vi "AlliGator Update Phasor Ratio Reference.vi"(7 "State Indicators Refnum":refnum<vi>, 8 "error in (no error)":errorcluster, 9 "Lifetime":dbl[unit], 10 "Reference Idx (0 or 1)":i32, 11 "Phasor":cluster{"X":dbl, "Y":dbl}) -> (0 "error out":errorcluster)   [LabVIEW 2021, in "AlliGator Phasor Graph.lvlib"]
doc: "Sets Phasor References status LEDs."
uses:
  AlliGator Phasor Graph.lvlib
  Globals, Variables, Constants/AlliGator Variables List.ctl
  Action Engine/AlliGator State Indicators List.ctl
  Globals, Variables, Constants/AlliGator Globals, Variables & Constants.lvlib
  Action Engine/AlliGator Action Engine.lvlib
  GUI/AlliGator GUI.lvlib
  Settings/AlliGator Settings.lvlib
  Error/Error.lvlib
panel:
  # "see the AlliGator License on the block diagram (Ctrl+E or Window:Show Block Diagram)"
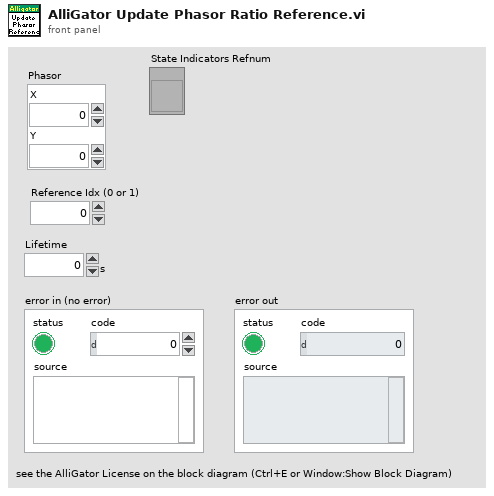
[diagram p1: front panel]
types:
  T1 = typedef "AlliGator Globals, Variables & Constants.lvlib/AlliGator Variables List.ctl" = enum16{"---- GUI ----", "GUI:Initialization Status", "GUI:State Indicators Refnum", "GUI:Original AlliGator Menu Items", "GUI:Current Action Loop State", "GUI:Script in progress", "GUI:Playback", "GUI:Loop Playback", "GUI:Search ROI Used", "GUI:Search ROI", "Decay Graph Max Legend Size", "Intensity Graph Max Legend Size", "Decay Statistics Graph Max Legend Size", "Phasor Graph Max Legend Size", "Phasor Ratio Graph Max Legend Size", "Lifetime Graph Max Legend Size", "---- Files ----", "Files:Export Dataset Frames as Individual Files", "Files:Show Batch Export Help Balloons", "Files:Frames in Dataset", "Files:ptu File Frame Start Indices", "Files:Current Frame in Dataset", "Files:Current Frame Timestamp", "Files:Dataset Loaded", "Files:Dataset Metadata", "Files:Dataset Channel", "Files:Dataset Data Description", "Files:Background Dataset Metadata", "Files:Background Dataset Channel", "Files:Background Dataset Data Description", "Files:Background File Subtraction", "Files:Background File Path", "Files:Background File Pile-up Correction", "Files:Background File Pixel Well Capacity", "Files:Background File Scaling Factor", "Files:Current Dataset Load Settings", "Files:Dataset Path", "Files:ICCD-specific Information", "Files:Macrotime Gate Separation", "------ Python Plugins ------", "Python Plugins:Information", "Python Plugins:Python Session", "Python Plugins:Valid Python Session?", "---- Source Image ----", "Source Image:ROIs", "Source Image:Current ROI", "Source Image:ROI Event Refnum", "X_Source Image Display Range", "X_Source Image Palette Information", "X_Type of Displayed Image", "X_Time Gate Slider", "Source Image:Palette List", "Source Image:Scale", "Source Image:ROI Overlay Color", "Source Image:Overlay to Erase", "Source Image:Is Displayed Image Accumulated", "Source Image:White Light Image Modified", "Source Image:Mask Image Modified", "---- Image Profile Window ----", "Image Profile:Window Event Refnum", "Image Profile:IntensityType", "Image Profile:Intensity Average Type", "Image Profile:Intensity-weighted SDV", "Image Profile:Box Profile Type", "Image Profile:Window Open", "Image Profile:Plotted Fit Parameter", "------ Phasor Graph -------", "Phasor Graph:Show Line", "---- Phasor Plot ---", "Phasor Plot:Parameters Changed", "Phasor Plot:FLI Dataset Modified since last Calculation", "Phasor Harmonics Data", "Selected Phasor Harmonics", "Phasor Harmonic Manager Event Refnum", "Phasor Plot:ROIs", "Phasor Plot:Current ROI", "Phasor Plot:ROI Event Refnum", "Phasor Plot:Image Reference Points", "Phasor Plot:Computed", "Phasor Plot:Palette Information", "Phasor Plot:Palette List", "Phasor Plot:Phasor Ratio Palette Information", "Phasor Plot:Phasor Ratio Palette List", "Phasor Plot:Image Scale", "Phasor Plot:Image Overlay to Erase", "Phasor Plot:Image Elements to Update", "Phasor Plot:Current Calculation Parameters", "Phasor Plot:Current Calibration Options", "Phasor Plot:Reset Cumulated Phasor Plot", "Phasor Plot:Reference 1", "Phasor Plot:Lifetime Reference 1", "Phasor Plot:Reference 1 Frequency", "Phasor Plot:Reference 2", "Phasor Plot:Lifetime Reference 2", "Phasor Plot:Reference 2 Frequency", "---- Decay Analysis ----", "Number of Selected Decays to Fit", "LS Fit Results", "LAR Fit Results", "BS Fit Results", "Last Decay Max - Min", "Best Fit Parameters", "Best Fit Parameter Names", "Actual Size X", "Actual Size Y", "Binning X", "Binning Y", "Actual # Gates", "Dataset Number", "Gates to...", "Gates Skipped", "Gates to keep", "Gate Step", "Gate Separation", "Reversed Gates", "Pile-up Correction", "Pixel Well Capacity", "Background Subtracted", "Background Subtraction Method", "Background Definition Range", "Background File (deprecated)", "Number of Dataset Accumulated", "Array of Accumulated Dataset Paths", "Do Averaged Datasets", "Destination File Path", "Process Plot Target", "Use 1/D as Phasor Frequency", "---- Decay Fit Parameter Map -----", "Decay Fit Parameter Map:Palette Information", "Decay Fit Parameter Map:Palette List", "---- Parameter Map ----", "Parameter Map:Palette Information", "Parameter Map:Palette List", "------- Local Decay Window ---------", "Local Decay Graph Window:Event Refnum", "Local Decay Graph Window:Use normalized IRF for convolution", "----- Miscellaneous ----", "Misc:Skippable Dialog Windows Status"}
  T2 = typedef "AlliGator Action Engine.lvlib/AlliGator State Indicators List.ctl" = enum16{"Phasor Calibration Defined", "Phasor Calibration Series Defined", "Phasor Calibration Map Defined", "Phasor Reference 1 Defined", "Phasor Reference 2 Defined", "Lifetime Reference 1 Defined", "Lifetime Reference 2 Defined", "Phasor Calibration Used", "Phasor Calibration Series Used", "Phasor Calibration Map Used", "Dataset Update Needed", "Phasor Plot Update Needed", "Reference/IRF Defined", "Individual IRFs Defined"}
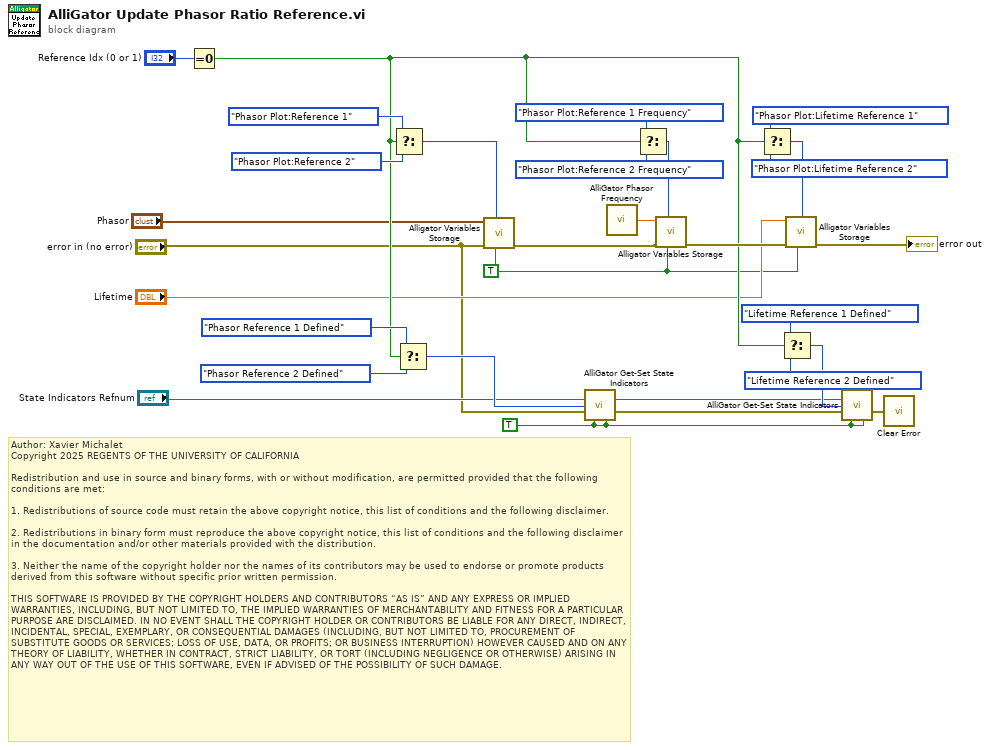
[diagram p0: block diagram]
diagram:
  w2 = TRUE ("Get(F)/Set")
  w1 = TRUE ("Set (T)/Unset (F)")
  # "Author: Xavier Michalet\nCopyright 2025 REGENTS OF THE UNIVERSITY OF CALIFORNIA\n\nRedistribution and use in source and binary forms, with or without modification, are permitted provided that the following conditions are met:\n\n1. Redistributions of source code must retain the above copyright notice, this list of conditions and the following disclaimer.\n\n2. Redistributions in binary form must reproduce the above copyright notice, this list of conditions and the following disclaimer in the documentation and/or other materials provided with the distribution.\n\n3. Neither the name of the copyright holder nor the names of its contributors may be used to endorse or promote products derived from this software without specific prior written permission.\n\nTHIS SOFTWARE IS PROVIDED BY THE COPYRIGHT HOLDERS AND CONTRIBUTORS “AS IS” AND ANY EXPRESS OR IMPLIED WARRANTIES, INCLUDING, BUT NOT LIMITED TO, THE IMPLIED WARRANTIES OF MERCHANTABILITY AND FITNESS FOR A PARTICULAR PURPOSE ARE DISCLAIMED. IN NO EVENT SHALL THE COPYRIGHT HOLDER OR CONTRIBUTORS BE LIABLE FOR ANY DIRECT, INDIRECT, INCIDENTAL, SPECIAL, EXEMPLARY, OR CONSEQUENTIAL DAMAGES (INCLUDING, BUT NOT LIMITED TO, PROCUREMENT OF SUBSTITUTE GOODS OR SERVICES; LOSS OF USE, DATA, OR PROFITS; OR BUSINESS INTERRUPTION) HOWEVER CAUSED AND ON ANY THEORY OF LIABILITY, WHETHER IN CONTRACT, STRICT LIABILITY, OR TORT (INCLUDING NEGLIGENCE OR OTHERWISE) ARISING IN ANY WAY OUT OF THE USE OF THIS SOFTWARE, EVEN IF ADVISED OF THE POSSIBILITY OF SUCH DAMAGE."
  n1 = Equal To 0?(x="Reference Idx (0 or 1)") -> (x = 0?=w10:bool)
  n2 = Select(t=AlliGator_Variables_List."Phasor Plot:Reference 1" ("Alligator Variable"), s=w10, f=AlliGator_Variables_List."Phasor Plot:Reference 2" ("Alligator Variable")) -> (s? t:f=w14:T1)
  n3 = Select(t=AlliGator_State_Indicators_List."Phasor Reference 1 Defined" ("Time-Gated Phasor Analysis Task List"), s=w10, f=AlliGator_State_Indicators_List."Phasor Reference 2 Defined" ("Time-Gated Phasor Analysis Task List")) -> (s? t:f=w21:T2)
  n4 = call "Alligator Variables Storage.vi"("Get(F)/Set"=w2, "AlliGator Variable"=w14, "Error In"="error in (no error)", "Data in"="Phasor") -> ("Error Out"=w3:errorcluster)  [unwired: 5 in, 2 out]
  n5 = call "AlliGator Get-Set State Indicators.vi"("State Indicators Refnum"="State Indicators Refnum", "AlliGator State Indicators List"=w21, "Error In"="error in (no error)", "ON/OFF"=w1, "Set (T)/Get"=w1) -> ("Error Out"=w7:errorcluster)  [unwired: 8 in, 2 out]
  n6 = call "AlliGator Phasor Frequency.vi"() -> ("Phasor Frequency"=w29:dbl[unit])
  n7 = Select(t=AlliGator_Variables_List."Phasor Plot:Reference 1 Frequency" ("Alligator Variable"), s=w10, f=AlliGator_Variables_List."Phasor Plot:Reference 2 Frequency" ("Alligator Variable")) -> (s? t:f=w28:T1)
  n8 = call "Alligator Variables Storage.vi"("Get(F)/Set"=w2, "AlliGator Variable"=w28, "Error In"=w3, "Data in"=w29) -> ("Error Out"=w25:errorcluster)  [unwired: 5 in, 2 out]
  n9 = Select(t=AlliGator_Variables_List."Phasor Plot:Lifetime Reference 1" ("Alligator Variable"), s=w10, f=AlliGator_Variables_List."Phasor Plot:Lifetime Reference 2" ("Alligator Variable")) -> (s? t:f=w17:T1)
  n10 = Select(t=AlliGator_State_Indicators_List."Lifetime Reference 1 Defined" ("Time-Gated Phasor Analysis Task List"), s=w10, f=AlliGator_State_Indicators_List."Lifetime Reference 2 Defined" ("Time-Gated Phasor Analysis Task List")) -> (s? t:f=w23:T2)
  n11 = call "Alligator Variables Storage.vi"("Get(F)/Set"=w2, "AlliGator Variable"=w17, "Error In"=w25, "Data in"="Lifetime") -> ("Error Out"=→"error out":errorcluster)  [unwired: 5 in, 2 out]
  n12 = call "AlliGator Get-Set State Indicators.vi"("State Indicators Refnum"="State Indicators Refnum", "AlliGator State Indicators List"=w23, "Error In"=w7, "ON/OFF"=w1, "Set (T)/Get"=w1) -> ("Error Out"=w5:errorcluster)  [unwired: 8 in, 2 out]
  n13 = call "Clear Error.vi"("Error In"=w5) -> ()  [unwired: 8 in, 1 out]
